vi "loadSummary.vi"(9 "machine":string, 11 "path":path) -> (0 "error out":errorcluster)   [LabVIEW 2012]
uses:
  <vilib>/addons/database/Auxilliary.llb/DB Tools Cursor Type.ctl
  <vilib>/addons/database/Connection.llb/DB Tools Open Connec (Path).vi
  <vilib>/addons/database/Connection.llb/Conn Execute.vi
  <vilib>/addons/database/Recordset.llb/Rec Destroy - Connection.vi
  <vilib>/addons/database/NI_Database_API.lvlib
panel:
  out "after substring":string
  out "concatenated string":string
  out "output cluster":T1
  in  "input cluster 2":T1
  out "filenames":string[](array[string])
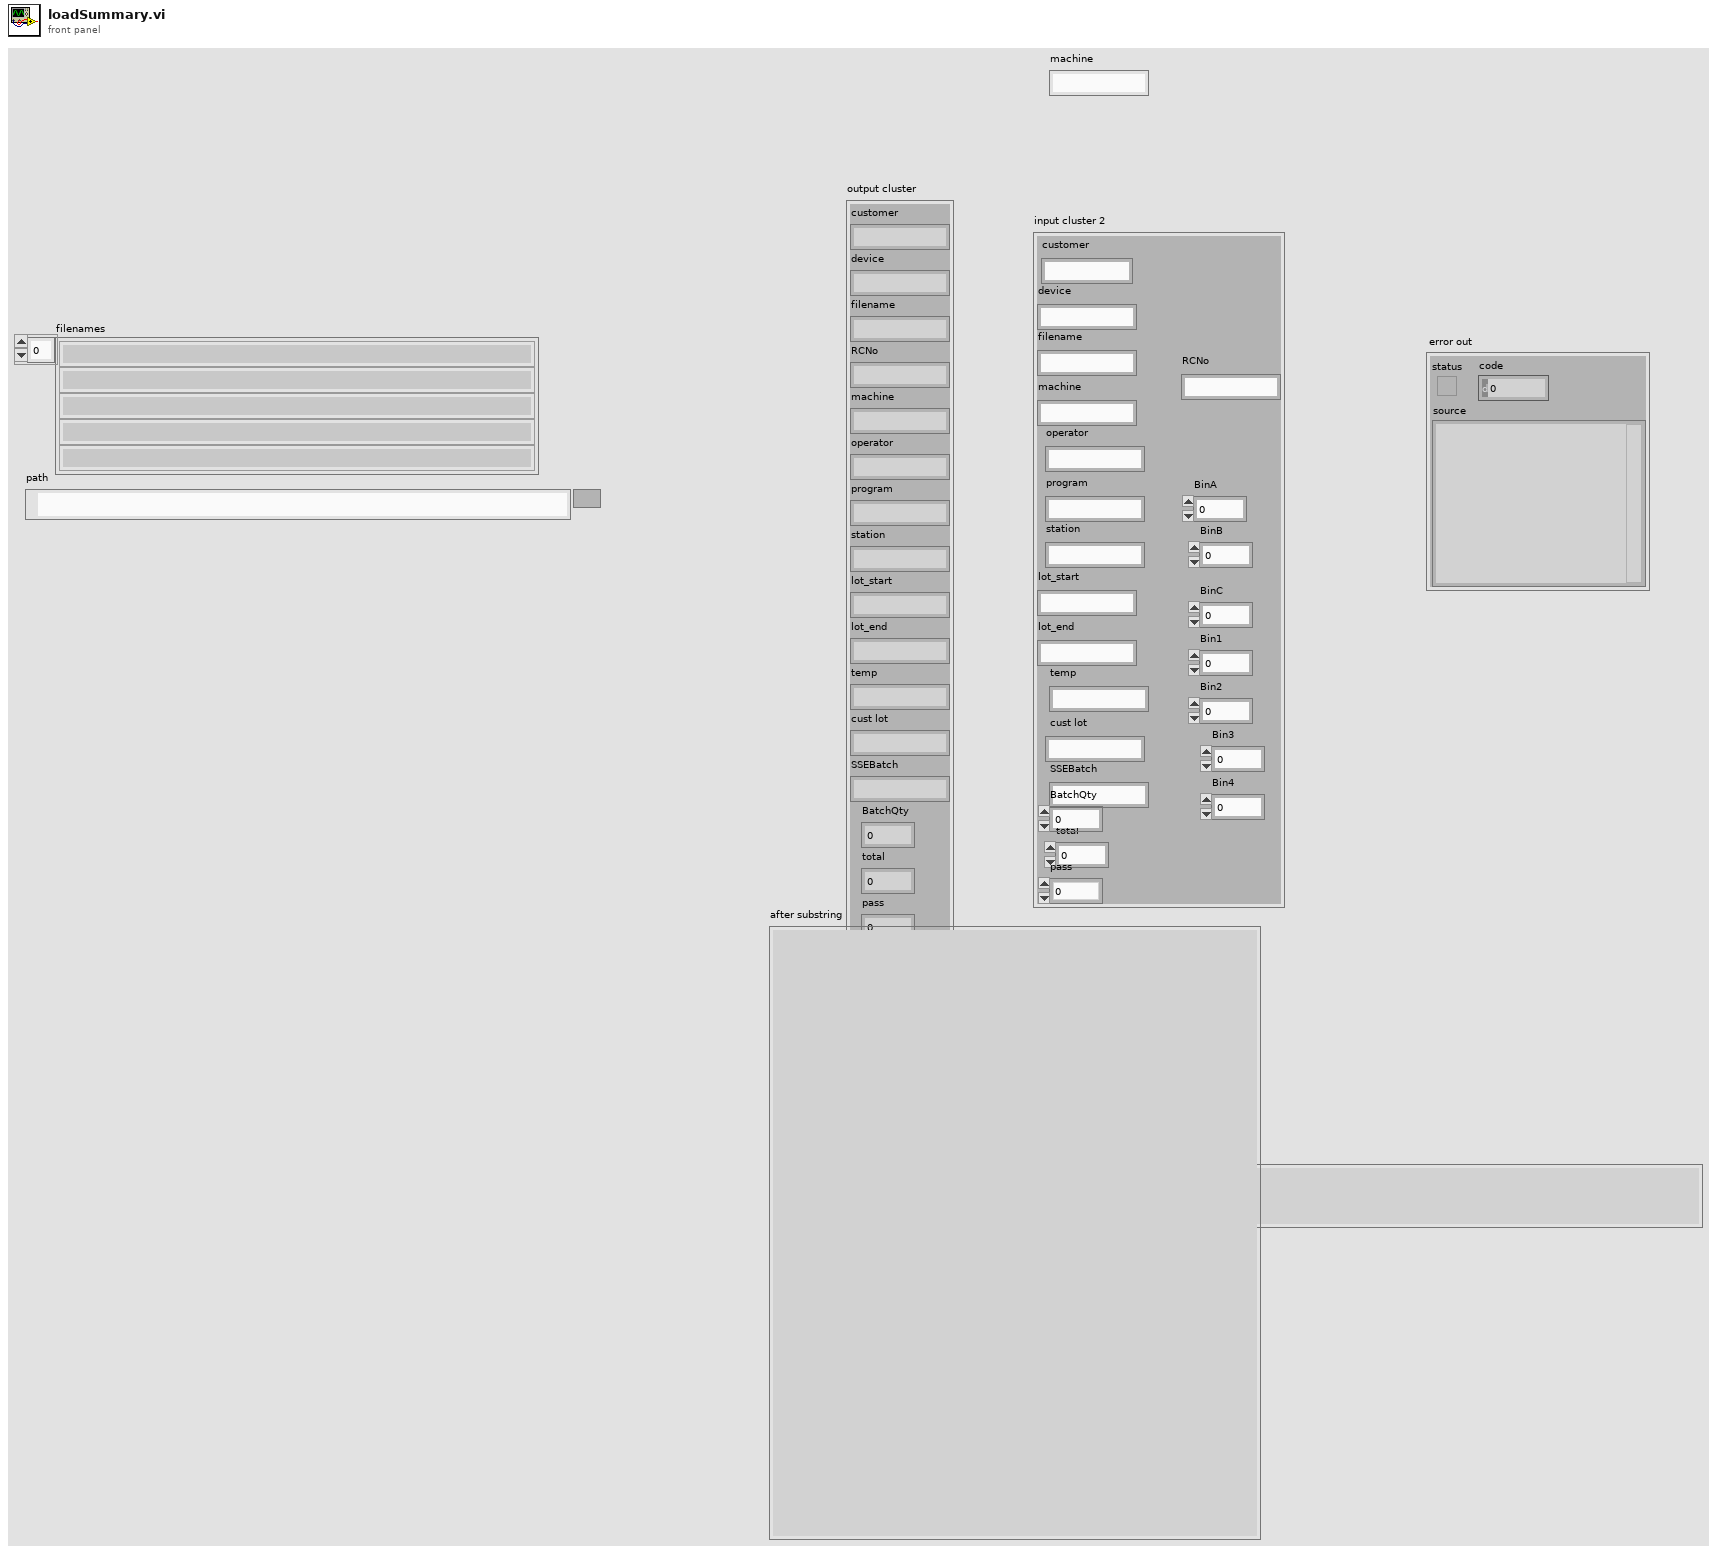
[diagram p1: front panel]
types:
  T1 = cluster{"customer":string, "device":string, "filename":string, "RCNo":string, "machine":string, "operator":string, "program":string, "station":string, "lot_start":string, "lot_end":string, "temp":string, "cust lot":string, "SSEBatch":string, "BatchQty":dbl, "total":dbl, "pass":dbl, "BinA":dbl, "BinB":dbl, "BinC":dbl, "Bin1":dbl, "Bin2":dbl, "Bin3":dbl, "Bin4":dbl}
  T2 = typedef "NI_Database_API.lvlib/Conn ObjectReference.ctl" = refnum<k1>
  T3 = typedef "NI_Database_API.lvlib/DB Tools Cursor Type.ctl" = enum16{"forward-only", "keyset", "dynamic", "static"}
  T4 = typedef "NI_Database_API.lvlib/Rec ObjectReference.ctl" = refnum<k1>
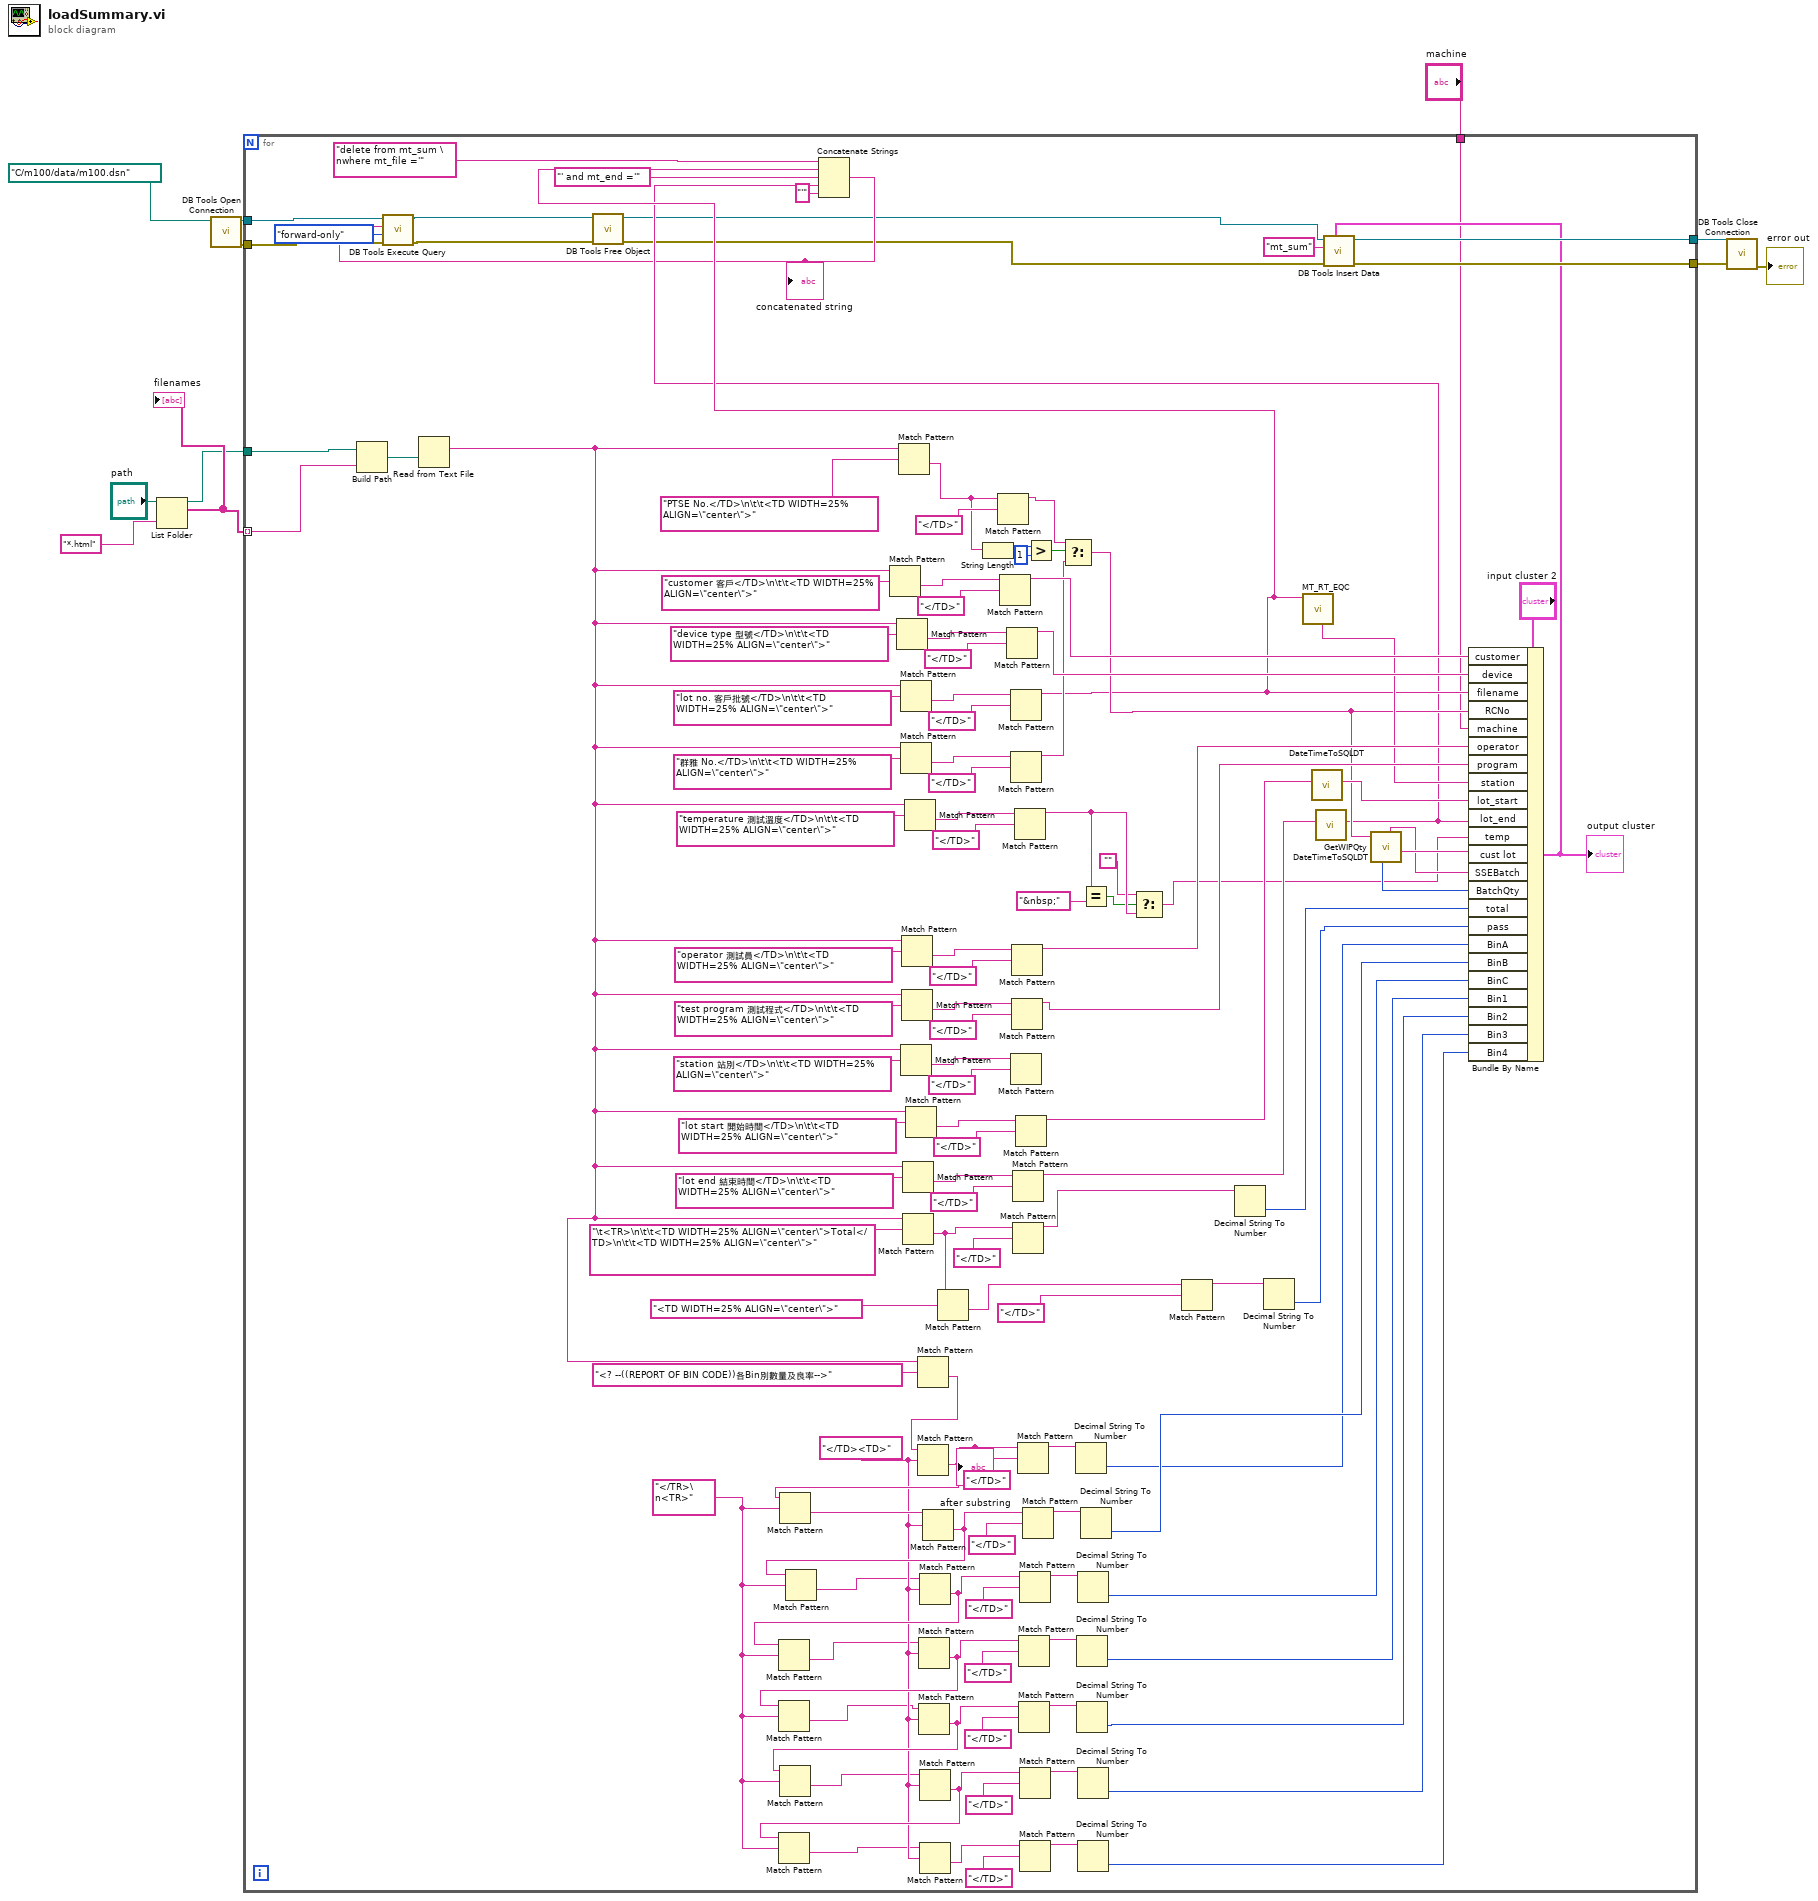
[diagram p0: block diagram]
diagram:
  n1 = List Folder(path="path", pattern="*.html") -> (path out=w9:path, filenames=w10:string[])  [unwired: 2 in, 2 out]
  "filenames" <- w10
  n2 = call-poly <vilib>:"DB Tools Open Connection.vi"("connection information"=path "C:/m100/data/m100.dsn") -> ("error out"=w5:errorcluster, "connection reference"=w6:T2)  [unwired: 7 in]
  n3 = for {
    tunnel: w10 -> [w136] mode=indexing
    tunnel: w9 -> [w135]
    tunnel: w6 -> [w48]
    tunnel: w5 -> [w47]
    tunnel: [w68] -> w4
    tunnel: [w67] -> w3
    tunnel: "machine" -> [w37]
    w26 = "</TR>\n<TR>" ("regular expression")
    w25 = "</TD><TD>" ("regular expression")
    n4 = Build Path(base path=w135, name or relative path=w136) -> (appended path=w137:path)
    n5 = Read from Text File(file (use dialog)=w137) -> (text=w35:string)  [unwired: 3 in, 3 out]
    n6 = Match Pattern(string=w35, regular expression="customer 客戶</TD>\n\t\t<TD WIDTH=25% ALIGN=\"center\">") -> (after substring=w133:string)  [unwired: 1 in, 3 out]
    n7 = Match Pattern(string=w35, regular expression="device type 型號</TD>\n\t\t<TD WIDTH=25% ALIGN=\"center\">") -> (after substring=w130:string)  [unwired: 1 in, 3 out]
    n8 = Match Pattern(string=w35, regular expression="PTSE No.</TD>\n\t\t<TD WIDTH=25% ALIGN=\"center\">") -> (after substring=w89:string)  [unwired: 1 in, 3 out]
    n9 = Match Pattern(string=w35, regular expression="lot no. 客戶批號</TD>\n\t\t<TD WIDTH=25% ALIGN=\"center\">") -> (after substring=w127:string)  [unwired: 1 in, 3 out]
    n10 = Match Pattern(string=w35, regular expression="群雅 No.</TD>\n\t\t<TD WIDTH=25% ALIGN=\"center\">") -> (after substring=w124:string)  [unwired: 1 in, 3 out]
    n11 = Match Pattern(string=w35, regular expression="station 站別</TD>\n\t\t<TD WIDTH=25% ALIGN=\"center\">") -> (after substring=w112:string)  [unwired: 1 in, 3 out]
    n12 = Match Pattern(string=w35, regular expression="operator 測試員</TD>\n\t\t<TD WIDTH=25% ALIGN=\"center\">") -> (after substring=w118:string)  [unwired: 1 in, 3 out]
    n13 = Match Pattern(string=w35, regular expression="test program 測試程式</TD>\n\t\t<TD WIDTH=25% ALIGN=\"center\">") -> (after substring=w115:string)  [unwired: 1 in, 3 out]
    n14 = Match Pattern(string=w35, regular expression="lot end 結束時間</TD>\n\t\t<TD WIDTH=25% ALIGN=\"center\">") -> (after substring=w106:string)  [unwired: 1 in, 3 out]
    n15 = Match Pattern(string=w35, regular expression="\t<TR>\n\t\t<TD WIDTH=25% ALIGN=\"center\">Total</TD>\n\t\t<TD WIDTH=25% ALIGN=\"center\">") -> (after substring=w102:string)  [unwired: 1 in, 3 out]
    n16 = Match Pattern(string=w35, regular expression="temperature 測試溫度</TD>\n\t\t<TD WIDTH=25% ALIGN=\"center\">") -> (after substring=w121:string)  [unwired: 1 in, 3 out]
    n17 = Match Pattern(string=w35, regular expression="lot start 開始時間</TD>\n\t\t<TD WIDTH=25% ALIGN=\"center\">") -> (after substring=w109:string)  [unwired: 1 in, 3 out]
    n18 = Match Pattern(string=w35, regular expression="<? --((REPORT OF BIN CODE))各Bin別數量及良率-->") -> (after substring=w34:string)  [unwired: 1 in, 3 out]
    n19 = Match Pattern(string=w34, regular expression=w25) -> (after substring=w33:string)  [unwired: 1 in, 3 out]
    "after substring" <- w33
    n20 = Match Pattern(string=w33, regular expression=w26) -> (after substring=w32:string)  [unwired: 1 in, 3 out]
    n21 = Match Pattern(string=w32, regular expression=w25) -> (after substring=w31:string)  [unwired: 1 in, 3 out]
    n22 = Match Pattern(string=w31, regular expression=w26) -> (after substring=w24:string)  [unwired: 1 in, 3 out]
    n23 = Match Pattern(string=w24, regular expression=w25) -> (after substring=w30:string)  [unwired: 1 in, 3 out]
    n24 = Match Pattern(string=w30, regular expression=w26) -> (after substring=w23:string)  [unwired: 1 in, 3 out]
    n25 = Match Pattern(string=w23, regular expression=w25) -> (after substring=w29:string)  [unwired: 1 in, 3 out]
    n26 = Match Pattern(string=w29, regular expression=w26) -> (after substring=w22:string)  [unwired: 1 in, 3 out]
    n27 = Match Pattern(string=w22, regular expression=w25) -> (after substring=w28:string)  [unwired: 1 in, 3 out]
    n28 = Match Pattern(string=w28, regular expression=w26) -> (after substring=w21:string)  [unwired: 1 in, 3 out]
    n29 = Match Pattern(string=w21, regular expression=w25) -> (after substring=w27:string)  [unwired: 1 in, 3 out]
    n30 = Match Pattern(string=w27, regular expression=w26) -> (after substring=w20:string)  [unwired: 1 in, 3 out]
    n31 = Match Pattern(string=w20, regular expression=w25) -> (after substring=w70:string)  [unwired: 1 in, 3 out]
    n32 = Match Pattern(string=w102, regular expression="<TD WIDTH=25% ALIGN=\"center\">") -> (after substring=w99:string)  [unwired: 1 in, 3 out]
    n33 = String Length(string=w89) -> (length=w87:i32)
    n34 = Match Pattern(string=w89, regular expression="</TD>") -> (before substring=w85:string)  [unwired: 1 in, 3 out]
    n35 = Match Pattern(string=w133, regular expression="</TD>") -> (before substring=w96:string)  [unwired: 1 in, 3 out]
    n36 = Match Pattern(string=w130, regular expression="</TD>") -> (before substring=w95:string)  [unwired: 1 in, 3 out]
    n37 = Match Pattern(string=w127, regular expression="</TD>") -> (before substring=w45:string)  [unwired: 1 in, 3 out]
    n38 = Match Pattern(string=w124, regular expression="</TD>") -> (before substring=w84:string)  [unwired: 1 in, 3 out]
    n39 = Match Pattern(string=w112, regular expression="</TD>") -> ()  [unwired: 1 in, 4 out]
    n40 = Match Pattern(string=w118, regular expression="</TD>") -> (before substring=w94:string)  [unwired: 1 in, 3 out]
    n41 = Match Pattern(string=w115, regular expression="</TD>") -> (before substring=w93:string)  [unwired: 1 in, 3 out]
    n42 = Match Pattern(string=w106, regular expression="</TD>") -> (before substring=w64:string)  [unwired: 1 in, 3 out]
    n43 = Match Pattern(string=w102, regular expression="</TD>") -> (before substring=w98:string)  [unwired: 1 in, 3 out]
    n44 = Match Pattern(string=w121, regular expression="</TD>") -> (before substring=w17:string)  [unwired: 1 in, 3 out]
    n45 = Match Pattern(string=w109, regular expression="</TD>") -> (before substring=w66:string)  [unwired: 1 in, 3 out]
    n46 = Match Pattern(string=w33, regular expression="</TD>") -> (before substring=w82:string)  [unwired: 1 in, 3 out]
    n47 = Match Pattern(string=w29, regular expression="</TD>") -> (before substring=w76:string)  [unwired: 1 in, 3 out]
    n48 = Match Pattern(string=w28, regular expression="</TD>") -> (before substring=w74:string)  [unwired: 1 in, 3 out]
    n49 = Match Pattern(string=w30, regular expression="</TD>") -> (before substring=w78:string)  [unwired: 1 in, 3 out]
    n50 = Match Pattern(string=w27, regular expression="</TD>") -> (before substring=w72:string)  [unwired: 1 in, 3 out]
    n51 = Match Pattern(string=w70, regular expression="</TD>") -> (before substring=w69:string)  [unwired: 1 in, 3 out]
    n52 = Match Pattern(string=w31, regular expression="</TD>") -> (before substring=w80:string)  [unwired: 1 in, 3 out]
    n53 = Greater?(x=w87, y=1) -> (0:w88:bool)
    n54 = Select(t=w85, s=w88, f=w84) -> (s? t:f=w62:string)
    n55 = Decimal String To Number(string=w82) -> (number=w54:i32)  [unwired: 2 in, 1 out]
    n56 = Decimal String To Number(string=w76) -> (number=w57:i32)  [unwired: 2 in, 1 out]
    n57 = Decimal String To Number(string=w74) -> (number=w58:i32)  [unwired: 2 in, 1 out]
    n58 = Decimal String To Number(string=w78) -> (number=w56:i32)  [unwired: 2 in, 1 out]
    n59 = Decimal String To Number(string=w72) -> (number=w59:i32)  [unwired: 2 in, 1 out]
    n60 = Decimal String To Number(string=w69) -> (number=w60:i32)  [unwired: 2 in, 1 out]
    n61 = Equal?(x=w17, y="&nbsp;") -> (x = y?=w16:bool)
    n62 = Decimal String To Number(string=w80) -> (number=w55:i32)  [unwired: 2 in, 1 out]
    n63 = Select(t="", s=w16, f=w17) -> (s? t:f=w18:string)
    n64 = Match Pattern(string=w99, regular expression="</TD>") -> (before substring=w92:string)  [unwired: 1 in, 3 out]
    n65 = Decimal String To Number(string=w98) -> (number=w52:i32)  [unwired: 2 in, 1 out]
    n66 = Decimal String To Number(string=w92) -> (number=w53:i32)  [unwired: 2 in, 1 out]
    n67 = call "MT_RT_EQC.vi"("input string"=w45) -> ("STN"=w63:string)  [unwired: 6 in, 4 out]
    n68 = call "DateTimeToSQLDT.vi"("DateTimeString"=w66) -> ("SQLDateTime"=w65:string)  [unwired: 10 in]
    n69 = call "DateTimeToSQLDT.vi"("DateTimeString"=w64) -> ("SQLDateTime"=w43:string)  [unwired: 10 in]
    n70 = Concatenate Strings("delete from mt_sum \nwhere mt_file ='" ("SQL query"), w45, "' and mt_end ='" ("string"), w43, "'" ("string")) -> (w41:string)
    "concatenated string" <- w41
    n71 = call-poly <vilib>:"DB Tools Execute Query.vi"("error in (no error)"=w47, "cursor type"=DB_Tools_Cursor_Type."forward-only", "SQL query"=w41, "connection reference"=w48) -> ("error out"=w13:errorcluster, "recordset reference"=w14:T4)  [unwired: 4 in]
    n72 = call-poly <vilib>:"DB Tools Free Object.vi"("error in (no error)"=w13, "recordset reference"=w14) -> ("error out"=w38:errorcluster, "connection reference"=w39:T2)  [unwired: 8 in]
    n73 = call "GetWIPQty.vi"("Lotno"=w62) -> ("lotno"=w61:string, "SSEBATCH"=w50:string, "BATCHQTY"=w51:i32)  [unwired: 2 in, 6 out]
    n74 = Bundle By Name(cluster="input cluster 2", "customer"=w96, "device"=w95, "filename"=w45, "RCNo"=w62, "machine"=w37, "operator"=w94, "program"=w93, "station"=w63, "lot_start"=w65, "lot_end"=w43, "temp"=w18, "cust lot"=w61, "SSEBatch"=w50, "BatchQty"=w51, "total"=w52, "pass"=w53, "BinA"=w54, "BinB"=w55, "BinC"=w56, "Bin1"=w57, "Bin2"=w58, "Bin3"=w59, "Bin4"=w60) -> (w49:T1)
    "output cluster" <- w49
    n75 = call <vilib>:"DB Tools Insert Data.vi"("data"=w49, "error in (no error)"=w38, "table"="mt_sum", "connection reference"=w39) -> ("error out"=w67:errorcluster, "connection reference out"=w68:T2)  [unwired: 6 in]
  }
  n76 = call <vilib>:"DB Tools Close Connection.vi"("error in (no error)"=w3, "connection reference"=w4) -> ("error out"=→"error out":errorcluster)  [unwired: 5 in]
